vi "_Set_LO_frq_B10_WCA.vi"(1 "Bias_LO_equip":T1={"Node address"=19, "CAN Interface"="CAN0", "Cartridge band"=10, "Slave Node in"={"Address"=19, "Serial Number"=[16, 71, 55, 76, 1, 8, 0, -15]}, "ObjHandle out"=288096320, "POL"=0, "sb"=1, "GPIB_SM (SIS S,V)"="24", "GPIB_DMM (SIS I)"="22", "GPIB_SM (MAG I) "="25", "GPIB_SG(LO)"="19", "GPIB_PW (PAMP) "="6", "GPIB_TMP1(8ch)"="12", "GPIB_TMP2(2ch)  "="13", "WCA_avg"=10, "Rsen"=10.0, "BiasModule"=1, "LOModule "=2, "WCA_LO_FREQ_SET"={"YTO Low freq. [GHz]"=14.41, "YTO High freq. [GHz]"=17.71, "Kvco"=1, "Lock Pol."=0, "SET LO FREQ"=96.22222, "Multiplier"=6.0, "YTO (HEX)"=2015, "YTO ( FREQ)"=16.03381, "NULL PLL INTEGRATOR"=FALSE}, "Res for"=0} {"Res for" items=["none", "series res", "parallel res"]; "WCA_LO_FREQ_SET"."YTO ( FREQ)" min=25 max=150 step=0.0001 format="%.3f"; "WCA_LO_FREQ_SET"."Multiplier" min=3 max=6 step=3; "WCA_LO_FREQ_SET"."SET LO FREQ" min=25 max=150 step=0.0001 format="%.3f"; "WCA_LO_FREQ_SET"."Lock Pol." items=["Lower", "Upper"]; "WCA_LO_FREQ_SET"."Kvco" items=["7.5MHz/V", "15MHz/V"]; "WCA_LO_FREQ_SET"."YTO High freq. [GHz]" format="%.3f"; "WCA_LO_FREQ_SET"."YTO Low freq. [GHz]" format="%.3f"; "LOModule" items=["Manual Gunn+PAMP"=0, "PLL GUNN+PAMP"=5, "B10Lab LO"=1, "WCA LO"=2, ""=3, "YIG発信器"=4, "none"=99]; "BiasModule" items=["B10Lab Bias"=0, "WCA BiasModule"=1, "none"=99]; "Slave Node in"."Serial Number" format="%.0x"; "Slave Node in"."Address" format="%.0x"; "Cartridge band" max=10 step=1; "Node address" format="%.0x"}, 2 "LO_misc":T2={"LO FRQ(GHz)"=860.0, "LO multi "=9.0, "LocK?"=TRUE, "LO REF multi"=4.0, "wait (ms)"=100.0, "SG Pow Min (dBm)"=10.0, "SG Pow Max (dBm)"=20.0, "SG Pow Step (dBm)"=0.2, "SGPow OPT? "=TRUE, "SG set frq"=23.89638888888889, "SG set pow"=10.0}, 5 "error in (no error)":errorcluster) -> (14 "Bias_LO_equip 2":T1={"Node address"=19, "CAN Interface"="CAN0", "Cartridge band"=10, "Slave Node in"={"Address"=0, "Serial Number"=[]}, "ObjHandle out"=0, "POL"=1, "sb"=1, "GPIB_SM (SIS S,V)"="24", "GPIB_DMM (SIS I)"="22", "GPIB_SM (MAG I) "="25", "GPIB_SG(LO)"="19", "GPIB_PW (PAMP) "="6", "GPIB_TMP1(8ch)"="12", "GPIB_TMP2(2ch)  "="13", "WCA_avg"=10, "Rsen"=10.0, "BiasModule"=1, "LOModule "=1, "WCA_LO_FREQ_SET"={"YTO Low freq. [GHz]"=14.42, "YTO High freq. [GHz]"=17.7, "Kvco"=1, "Lock Pol."=0, "SET LO FREQ"=72.5, "Multiplier"=6.0, "YTO (HEX)"=0, "YTO ( FREQ)"=25.0, "NULL PLL INTEGRATOR"=FALSE}, "Res for"=0} {"Res for" items=["none", "series res", "parallel res"]; "WCA_LO_FREQ_SET"."YTO ( FREQ)" min=25 max=150 step=0.0001 format="%.4f"; "WCA_LO_FREQ_SET"."Multiplier" min=3 max=6 step=3; "WCA_LO_FREQ_SET"."SET LO FREQ" min=25 max=150 step=0.0001 format="%.3f"; "WCA_LO_FREQ_SET"."Lock Pol." items=["Lower", "Upper"]; "WCA_LO_FREQ_SET"."Kvco" items=["7.5MHz/V", "15MHz/V"]; "WCA_LO_FREQ_SET"."YTO High freq. [GHz]" format="%.3f"; "WCA_LO_FREQ_SET"."YTO Low freq. [GHz]" format="%.3f"; "LOModule" items=["Manual", "B10Lab LO", "WCA LO"]; "BiasModule" items=["B10Lab Bias", "WCA BiasModule"]; "Slave Node in"."Serial Number" format="%.0x"; "Slave Node in"."Address" format="%.0x"; "Cartridge band" max=10 step=1; "Node address" format="%.0x"}, 16 "LO_misc 2":T2={"LO FRQ(GHz)"=860.0, "LO multi "=9.0, "LocK?"=TRUE, "LO REF multi"=4.0, "wait (ms)"=100.0, "SG Pow Min (dBm)"=10.0, "SG Pow Max (dBm)"=20.0, "SG Pow Step (dBm)"=0.2, "SGPow OPT? "=TRUE, "SG set frq"=23.89638888888889, "SG set pow"=10.0}, 19 "error out":errorcluster)   [LabVIEW 2017]
uses:
  WCA_NAOJ_sub_vi/WCA_Global.vi
panel:
  # "LO freq. [GHz]"
  # "YTO LOW\n/High Freq."
  # "ZERO Intgrtr"
  # "Node Address"
  # "Serial Number"
  # "LO freq. [GHz]"
  # "YTO LOW\n/High Freq."
  # "ZERO Intgrtr"
  # "Node Address"
  # "Serial Number"
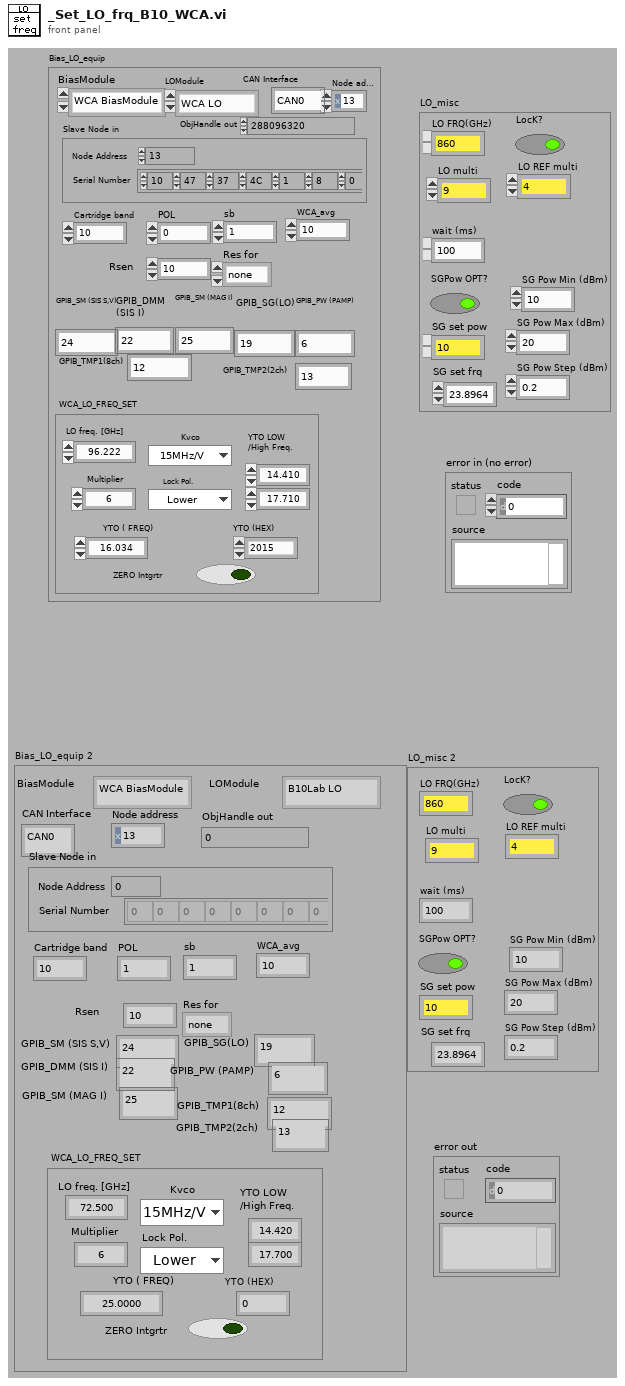
[diagram p1: front panel]
types:
  T1 = cluster{"Node address":u16, "CAN Interface":string, "Cartridge band":u32, "Slave Node in":cluster{"Address":i16, "Serial Number":i8[]}, "ObjHandle out":u32, "POL":u32, "sb":u32, "GPIB_SM (SIS S,V)":string, "GPIB_DMM (SIS I)":string, "GPIB_SM (MAG I) ":string, "GPIB_SG(LO)":string, "GPIB_PW (PAMP) ":string, "GPIB_TMP1(8ch)":string, "GPIB_TMP2(2ch)  ":string, "WCA_avg":i32, "Rsen":dbl, "BiasModule":u16, "LOModule ":u16, "WCA_LO_FREQ_SET":cluster{"YTO Low freq. [GHz]":sgl, "YTO High freq. [GHz]":sgl, "Kvco":u16, "Lock Pol.":u16, "SET LO FREQ":sgl, "Multiplier":sgl, "YTO (HEX)":u16, "YTO ( FREQ)":sgl, "NULL PLL INTEGRATOR":bool}, "Res for":u16}
  T2 = cluster{"LO FRQ(GHz)":dbl, "LO multi ":dbl, "LocK?":bool, "LO REF multi":dbl, "wait (ms)":dbl, "SG Pow Min (dBm)":dbl, "SG Pow Max (dBm)":dbl, "SG Pow Step (dBm)":dbl, "SGPow OPT? ":bool, "SG set frq":dbl, "SG set pow":dbl}
  T3 = cluster{"YTO Low freq. [GHz]":sgl, "YTO High freq. [GHz]":sgl, "Kvco":u16, "Lock Pol.":u16, "SET LO FREQ":sgl, "Multiplier":sgl, "YTO (HEX)":u16, "YTO ( FREQ)":sgl, "NULL PLL INTEGRATOR":bool}
  T4 = cluster{"YTO Low freq. [GHz]":sgl, "YTO High freq. [GHz]":sgl, "Kvco":u16, "Lock Pol.":u16, "SET LO FREQ":sgl, "Multiplier":sgl, "YTO coarse tune(HEX)":u16, "YTO coarse( FREQ)":sgl, "NULL PLL INTEGRATOR":bool}
  T5 = cluster{"PLL_ASSY_T":sgl, "PLL_REF_TOT_P":sgl, "PLL_IF_TOT_P":sgl, "PLL_CORR_V":sgl, "PLL_LOCK_V":sgl, "PLL_5V_SUPPLY_V":sgl, "Temp_TF":bool, "PLL Ref Pwr_TF":bool, "IF Pwr_TF":bool, "PLL Corr_TF":bool, "PLL Lock V_TF":bool, "PLL Nominal_TF":bool}
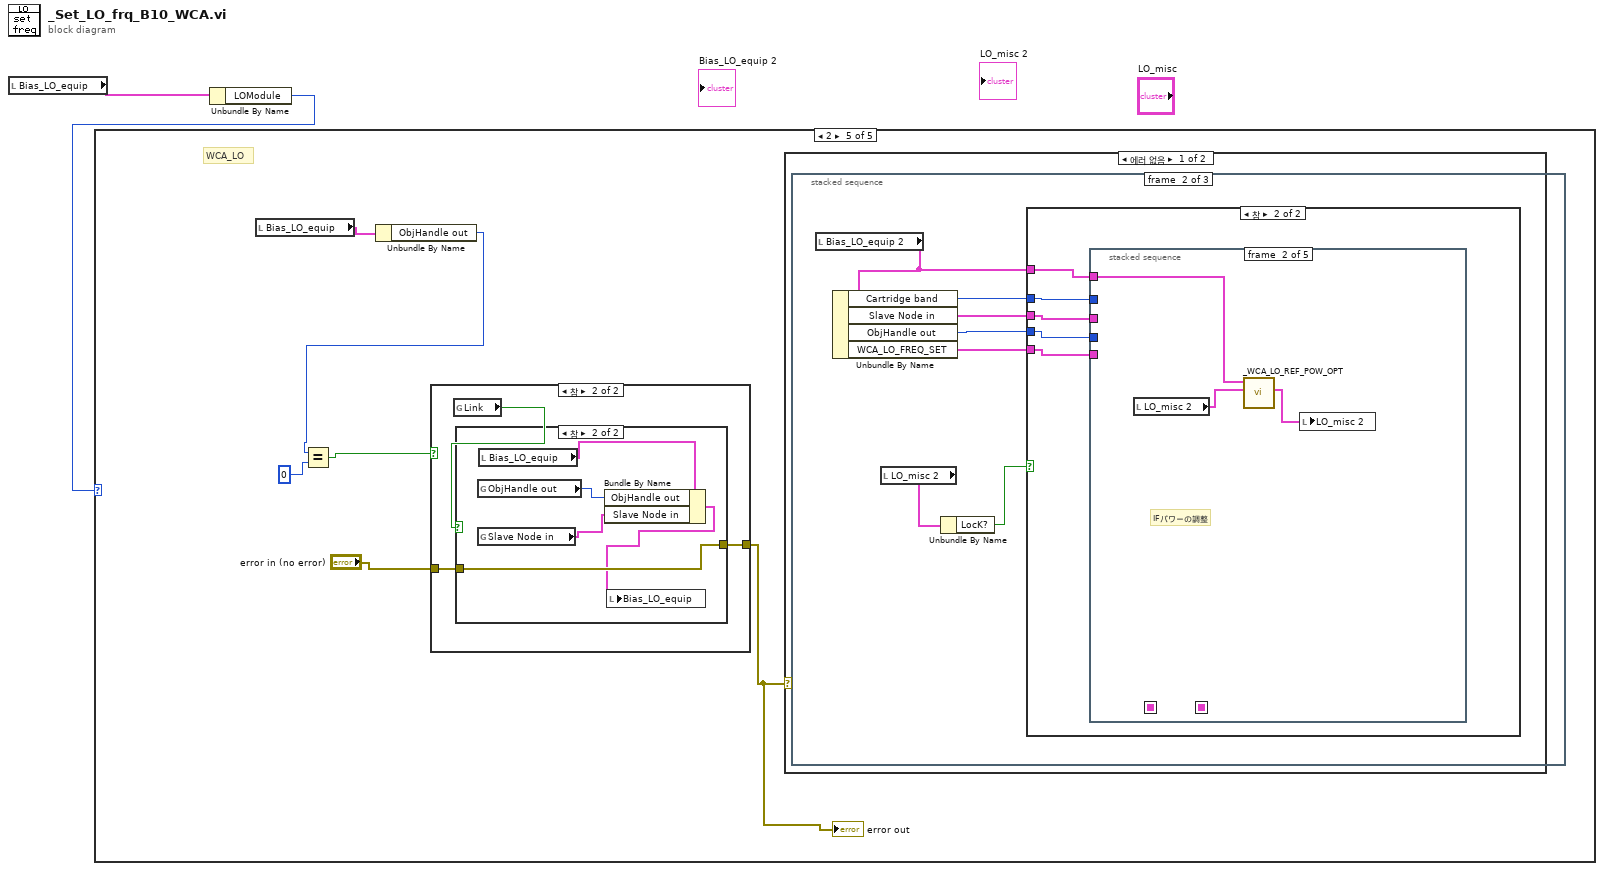
[diagram p0: block diagram]
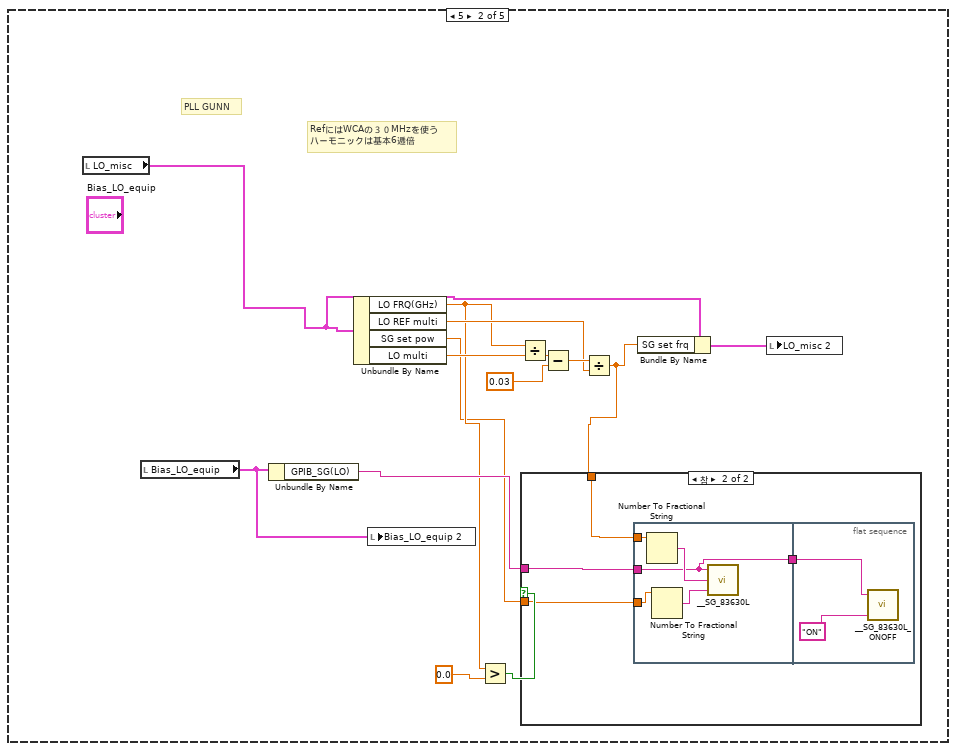
[diagram p3: hidden frame]
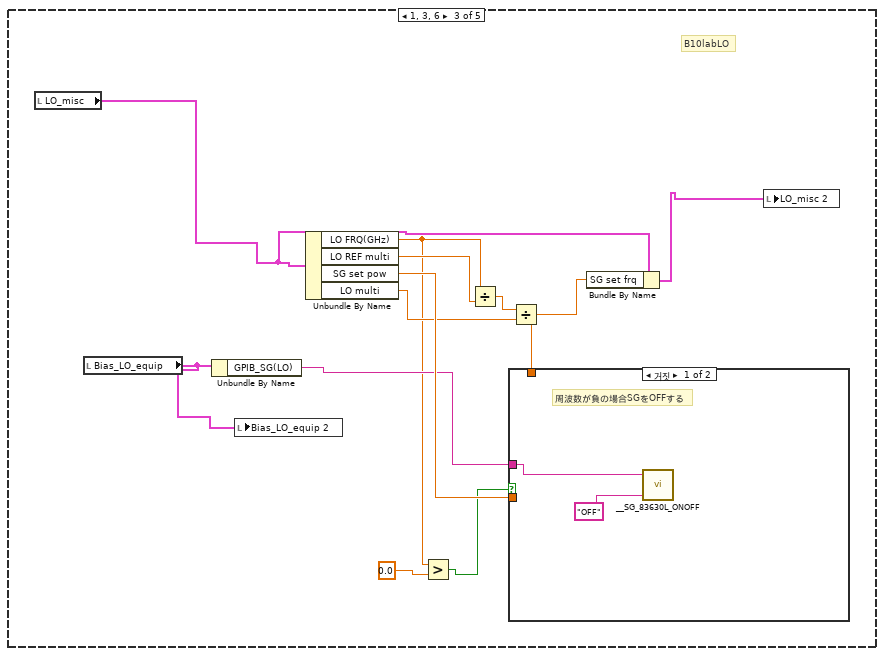
[diagram p5: hidden frame]
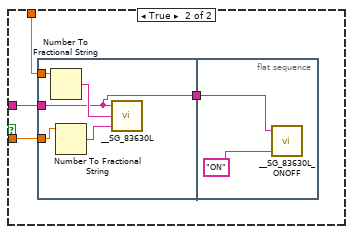
[diagram p6: hidden frame]
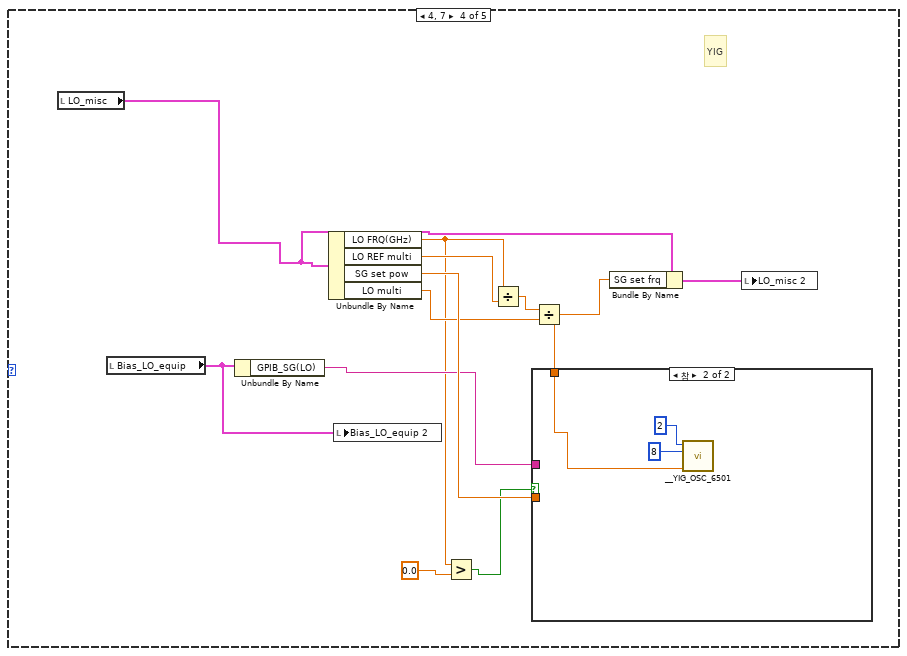
[diagram p7: hidden frame]
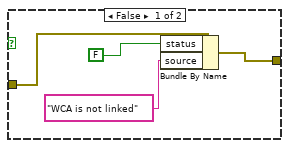
[diagram p10: hidden frame]
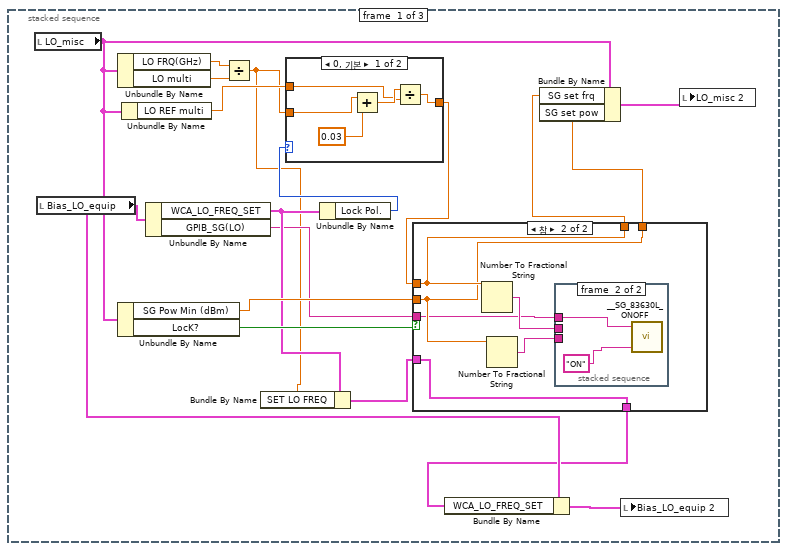
[diagram p11: hidden frame]
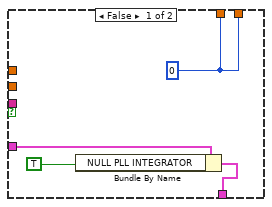
[diagram p12: hidden frame]
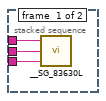
[diagram p13: hidden frame]
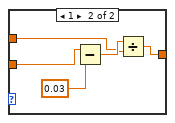
[diagram p14: hidden frame]
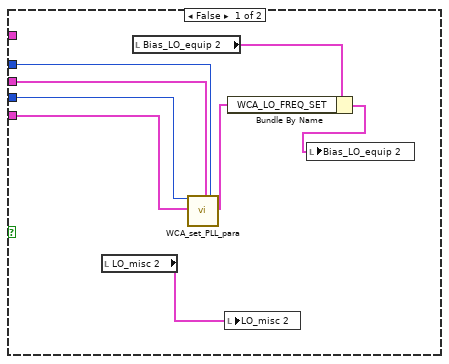
[diagram p15: hidden frame]
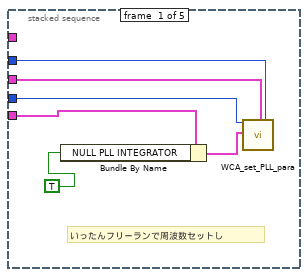
[diagram p16: hidden frame]
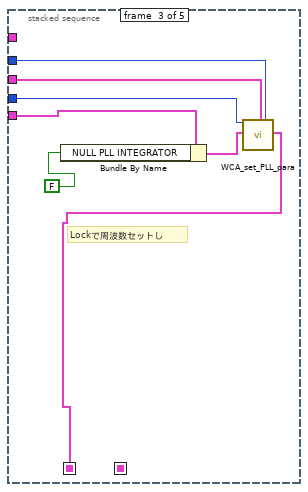
[diagram p17: hidden frame]
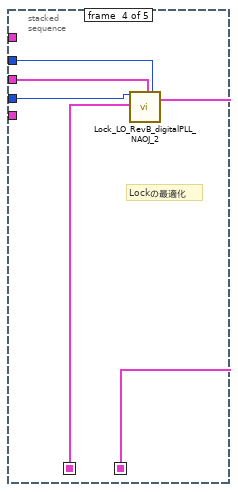
[diagram p18: hidden frame]
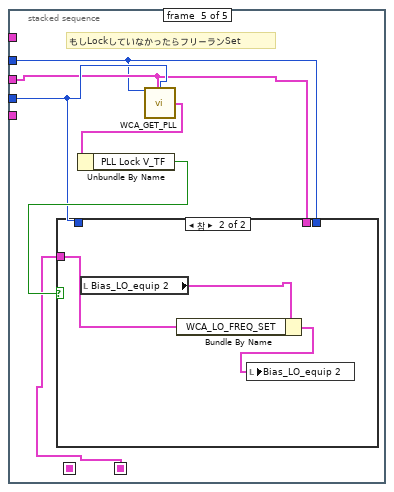
[diagram p19: hidden frame]
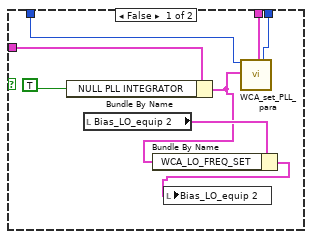
[diagram p20: hidden frame]
diagram:
  n1 = local read "Bias_LO_equip"() -> (w1:T1)
  n2 = Unbundle By Name(w1) -> ("LOModule"=w2:u16)
  n3 = case shown="2" w2 {
    frame 0, Default {
      # "Gunn unLock"
    }
    frame 5 {
      # "RefにはWCAの３０MHzを使う\nハーモニックは基本6逓倍"
      # "PLL GUNN"
      n4 = local read "LO_misc"() -> (w16:T2)
      n5 = local read "Bias_LO_equip"() -> (w6:T1)
      n6 = Unbundle By Name(w6) -> ("GPIB_SG(LO)"=w9:string)
      n7 = Unbundle By Name(w16) -> ("LO FRQ(GHz)"=w5:dbl, "LO REF multi"=w10:dbl, "SG set pow"=w3:dbl, "LO multi"=w14:dbl)
      n8 = local write "Bias_LO_equip 2"(w6) -> ()
      n9 = Greater?(x=w5, y=0.0) -> (0:w7:bool)
      n10 = Divide(x=w5, y=w14) -> (x/y=w13:dbl)
      n11 = Subtract(x=w13, y=0.03) -> (x-y=w11:dbl)
      n12 = Divide(x=w11, y=w10) -> (x/y=w4:dbl)
      n13 = case shown="참" w7 {
        tunnel: w3 -> [_ w17]
        tunnel: w4 -> [_ w18]
        tunnel: w9 -> [_ w19]
        frame False {
        }
        frame True {
          n14 = flat-sequence {
            tunnel: w18 -> [w24]
            tunnel: w17 -> [w22]
            tunnel: w19 -> [w21]
            tunnel: [w21] -> w20
            tunnel: w20 -> [w26]
            frame #0 {
              n15 = Number To Fractional String(number=w24) -> (F-format string=w25:string)  [unwired: 3 in]
              n16 = Number To Fractional String(number=w22) -> (F-format string=w23:string)  [unwired: 3 in]
              n17 = call "__SG_83630L.vi"("PW(dBm)"=w23, "frq(GHz)"=w25, "GPIB"=w21) -> ()
            }
            frame #1 {
              n18 = call "__SG_83630L_ONOFF.vi"("ON/OFF"="ON", "GPIB"=w26) -> ()  [unwired: 1 in]
            }
          }
        }
      }
      n19 = Bundle By Name(cluster=w16, "SG set frq"=w4) -> (w15:T2)
      n20 = local write "LO_misc 2"(w15) -> ()
    }
    frame 1, 3, 6 {
      # "B10labLO"
      n21 = local read "LO_misc"() -> (w30:T2)
      n22 = local read "Bias_LO_equip"() -> (w28:T1)
      n23 = Unbundle By Name(w28) -> ("GPIB_SG(LO)"=w34:string)
      n24 = local write "Bias_LO_equip 2"(w28) -> ()
      n25 = Unbundle By Name(w30) -> ("LO FRQ(GHz)"=w32:dbl, "LO REF multi"=w38:dbl, "SG set pow"=w37:dbl, "LO multi"=w35:dbl)
      n26 = Greater?(x=w32, y=0.0) -> (0:w31:bool)
      n27 = Divide(x=w32, y=w38) -> (x/y=w39:dbl)
      n28 = Divide(x=w39, y=w35) -> (x/y=w36:dbl)
      n29 = case shown="거짓" w31 {
        tunnel: w37 -> [_ w44]
        tunnel: w36 -> [_ w43]
        tunnel: w34 -> [w40 w42]
        frame False {
          # "周波数が負の場合SGをOFFする"
          n30 = call "__SG_83630L_ONOFF.vi"("ON/OFF"="OFF", "GPIB"=w40) -> ()  [unwired: 1 in]
        }
        frame True {
          n31 = flat-sequence {
            tunnel: w43 -> [w49]
            tunnel: w44 -> [w47]
            tunnel: w42 -> [w46]
            tunnel: [w46] -> w45
            tunnel: w45 -> [w51]
            frame #0 {
              n32 = Number To Fractional String(number=w49) -> (F-format string=w50:string)  [unwired: 3 in]
              n33 = Number To Fractional String(number=w47) -> (F-format string=w48:string)  [unwired: 3 in]
              n34 = call "__SG_83630L.vi"("PW(dBm)"=w48, "frq(GHz)"=w50, "GPIB"=w46) -> ()
            }
            frame #1 {
              n35 = call "__SG_83630L_ONOFF.vi"("ON/OFF"="ON", "GPIB"=w51) -> ()  [unwired: 1 in]
            }
          }
        }
      }
      n36 = Bundle By Name(cluster=w30, "SG set frq"=w36) -> (w29:T2)
      n37 = local write "LO_misc 2"(w29) -> ()
    }
    frame 4, 7 {
      # "YIG"
      n38 = local read "LO_misc"() -> (w55:T2)
      n39 = local read "Bias_LO_equip"() -> (w54:T1)
      n40 = Unbundle By Name(w54) -> ("GPIB_SG(LO)"=w59:string)
      n41 = Unbundle By Name(w55) -> ("LO FRQ(GHz)"=w57:dbl, "LO REF multi"=w63:dbl, "SG set pow"=w62:dbl, "LO multi"=w60:dbl)
      n42 = local write "Bias_LO_equip 2"(w54) -> ()
      n43 = Greater?(x=w57, y=0.0) -> (0:w56:bool)
      n44 = Divide(x=w57, y=w63) -> (x/y=w64:dbl)
      n45 = Divide(x=w64, y=w60) -> (x/y=w61:dbl)
      n46 = case shown="참" w56 {
        tunnel: w62 -> [_ _]
        tunnel: w61 -> [_ w65]
        tunnel: w59 -> [_ _]
        frame False {
        }
        frame True {
          n47 = call "__YIG_OSC_6501.vi"("fc(GHz)"=w65, "bit"=8, "Dev(1,2..)"=2) -> ()  [unwired: 1 in]
        }
      }
      n48 = Bundle By Name(cluster=w55, "SG set frq"=w61) -> (w53:T2)
      n49 = local write "LO_misc 2"(w53) -> ()
    }
    frame 2 {
      # "WCA_LO"
      n50 = local read "Bias_LO_equip"() -> (w70:T1)
      n51 = Unbundle By Name(w70) -> ("ObjHandle out"=w69:u32)
      n52 = Equal?(x=w69, y=0) -> (x = y?=w72:bool)
      n53 = case shown="참" w72 {
        tunnel: "error in (no error)" -> [w74 w77]
        tunnel: [w74 w76] -> w68
        frame False {
        }
        frame True {
          n54 = global read "WCA_Global.vi" "Link"() -> (w75:bool)
          n55 = case shown="참" w75 {
            tunnel: w77 -> [w81 w86]
            tunnel: [w78 w86] -> w76
            frame False {
              n56 = Bundle By Name(cluster=w81, "status"=FALSE, "source"="WCA is not linked") -> (w78:errorcluster)
            }
            frame True {
              n57 = global read "WCA_Global.vi" "ObjHandle out"() -> (w83:u32)
              n58 = global read "WCA_Global.vi" "Slave Node in"() -> (w84:cluster{"Address":i16, "Serial Number":i8[]})
              n59 = local read "Bias_LO_equip"() -> (w85:T1)
              n60 = Bundle By Name(cluster=w85, "ObjHandle out"=w83, "Slave Node in"=w84) -> (w82:T1)
              n61 = local write "Bias_LO_equip"(w82) -> ()
            }
          }
        }
      }
      "error out" <- w68
      n62 = case shown="에러 없음" w68 {
        frame No Error {
          n63 = stacked-sequence {
            frame #0 {
              n64 = local read "LO_misc"() -> (w103:T2)
              n65 = local read "Bias_LO_equip"() -> (w91:T1)
              n66 = Unbundle By Name(w103) -> ("LO FRQ(GHz)"=w101:dbl, "LO multi"=w102:dbl)
              n67 = Unbundle By Name(w103) -> ("SG Pow Min (dBm)"=w97:dbl, "LocK?"=w96:bool)
              n68 = Unbundle By Name(w103) -> ("LO REF multi"=w100:dbl)
              n69 = Unbundle By Name(w91) -> ("WCA_LO_FREQ_SET"=w94:T3, "GPIB_SG(LO)"=w93:string)
              n70 = Divide(x=w101, y=w102) -> (x/y=w92:dbl)
              n71 = Bundle By Name(cluster=w94, "SET LO FREQ"=w92) -> (w95:T3)
              n72 = Unbundle By Name(w94) -> ("Lock Pol."=w99:u16)
              n73 = case shown="0, 기본" w99 {
                tunnel: w92 -> [w124 w129]
                tunnel: w100 -> [w121 w126]
                tunnel: [w120 w125] -> w98
                frame 0, Default {
                  n74 = Add(x=w124, y=0.03) -> (x+y=w122:dbl)
                  n75 = Divide(x=w122, y=w121) -> (x/y=w120:dbl)
                }
                frame 1 {
                  n76 = Subtract(x=w129, y=0.03) -> (x-y=w127:dbl)
                  n77 = Divide(x=w127, y=w126) -> (x/y=w125:dbl)
                }
              }
              n78 = case shown="참" w96 {
                tunnel: w98 -> [_ w111]
                tunnel: w97 -> [_ w110]
                tunnel: w93 -> [_ w109]
                tunnel: w95 -> [w108 w112]
                tunnel: [w107 w112] -> w90
                tunnel: [w105 w111] -> w88
                tunnel: [w105 w110] -> w87
                frame False {
                  w105 = 0
                  n79 = Bundle By Name(cluster=w108, "NULL PLL INTEGRATOR"=TRUE) -> (w107:T3)
                }
                frame True {
                  n80 = Number To Fractional String(number=w111) -> (F-format string=w113:string)  [unwired: 3 in]
                  n81 = Number To Fractional String(number=w110) -> (F-format string=w114:string)  [unwired: 3 in]
                  n82 = stacked-sequence {
                    tunnel: w114 -> [w117 _]
                    tunnel: w113 -> [w116 _]
                    tunnel: w109 -> [w115 w119]
                    frame #0 {
                      n83 = call "__SG_83630L.vi"("PW(dBm)"=w117, "frq(GHz)"=w116, "GPIB"=w115) -> ()
                    }
                    frame #1 {
                      n84 = call "__SG_83630L_ONOFF.vi"("ON/OFF"="ON", "GPIB"=w119) -> ()  [unwired: 1 in]
                    }
                  }
                }
              }
              n85 = Bundle By Name(cluster=w91, "WCA_LO_FREQ_SET"=w90) -> (w89:T1)
              n86 = Bundle By Name(cluster=w103, "SG set frq"=w88, "SG set pow"=w87) -> (w104:T2)
              n87 = local write "Bias_LO_equip 2"(w89) -> ()
              n88 = local write "LO_misc 2"(w104) -> ()
            }
            frame #1 {
              n89 = local read "Bias_LO_equip 2"() -> (w130:T1)
              n90 = Unbundle By Name(w130) -> ("Cartridge band"=w132:u32, "Slave Node in"=w134:cluster{"Address":i16, "Serial Number":i8[]}, "ObjHandle out"=w133:u32, "WCA_LO_FREQ_SET"=w131:T3)
              n91 = local read "LO_misc 2"() -> (w135:T2)
              n92 = Unbundle By Name(w135) -> ("LocK?"=w136:bool)
              n93 = case shown="참" w136 {
                tunnel: w134 -> [w144 w147]
                tunnel: w133 -> [w141 w148]
                tunnel: w132 -> [w143 w146]
                tunnel: w131 -> [w142 w149]
                tunnel: w130 -> [_ w145]
                frame False {
                  n94 = local read "LO_misc 2"() -> (w137:T2)
                  n95 = local read "Bias_LO_equip 2"() -> (w140:T1)
                  n96 = call "WCA_set_PLL_para.vi"("ObjHandle in"=w141, "LO_FREQ_SET"=w142, "Slave Node in"=w144, "Cartridge band"=w143) -> ("LO_FREQ_SET output"=w138:T4)  [unwired: 14 in, 1 out]
                  n97 = local write "LO_misc 2"(w137) -> ()
                  n98 = Bundle By Name(cluster=w140, "WCA_LO_FREQ_SET"=w138) -> (w139:T1)
                  n99 = local write "Bias_LO_equip 2"(w139) -> ()
                }
                frame True {
                  n100 = stacked-sequence {
                    seq-local: [_ _ w159 _ _] -> [_ _ _ w170 _]
                    seq-local: [_ _ _ w166 _] -> [_ _ _ _ w171]
                    tunnel: w149 -> [w155 _ w165 _ _]
                    tunnel: w148 -> [w152 _ w162 w169 w174]
                    tunnel: w147 -> [w151 _ w161 w168 w173]
                    tunnel: w146 -> [w150 _ w160 w167 w172]
                    tunnel: w145 -> [_ w156 _ _ _]
                    frame #0 {
                      # "いったんフリーランで周波数セットし"
                      n101 = Bundle By Name(cluster=w155, "NULL PLL INTEGRATOR"=TRUE) -> (w153:T3)
                      n102 = call "WCA_set_PLL_para.vi"("ObjHandle in"=w152, "LO_FREQ_SET"=w153, "Slave Node in"=w151, "Cartridge band"=w150) -> ()  [unwired: 14 in, 2 out]
                    }
                    frame #1 {
                      # "IFパワーの調整"
                      n103 = local read "LO_misc 2"() -> (w158:T2)
                      n104 = call "_WCA_LO_REF_POW_OPT.vi"("LO_misc"=w158, "Bias_LO_equip"=w156) -> ("LO_misc 2"=w157:T2)  [unwired: 6 in, 1 out]
                      n105 = local write "LO_misc 2"(w157) -> ()
                    }
                    frame #2 {
                      # "Lockで周波数セットし"
                      n106 = Bundle By Name(cluster=w165, "NULL PLL INTEGRATOR"=FALSE) -> (w163:T3)
                      n107 = call "WCA_set_PLL_para.vi"("ObjHandle in"=w162, "LO_FREQ_SET"=w163, "Slave Node in"=w161, "Cartridge band"=w160) -> ("LO_FREQ_SET output"=w159:T4)  [unwired: 14 in, 1 out]
                    }
                    frame #3 {
                      # "Lockの最適化"
                      n108 = call "Lock_LO_RevB_digitalPLL_NAOJ_2.vi"("ObjHandle in"=w169, "LO_FREQ_SET"=w170, "Slave Node in"=w168, "Cartridge band"=w167) -> ("LO_FREQ_output"=w166:T4)  [unwired: 12 in, 3 out]
                    }
                    frame #4 {
                      # "もしLockしていなかったらフリーランSet"
                      n109 = call "WCA_GET_PLL.vi"("Cartridge Band"=w172, "Slave Node in"=w173, "ObjHandle in"=w174) -> ("GET_PLL"=w176:T5)  [unwired: 10 in, 2 out]
                      n110 = Unbundle By Name(w176) -> ("PLL Lock V_TF"=w175:bool)
                      n111 = case shown="참" w175 {
                        tunnel: w171 -> [w183 w185]
                        tunnel: w174 -> [w182 _]
                        tunnel: w173 -> [w181 _]
                        tunnel: w172 -> [w180 _]
                        frame False {
                          n112 = Bundle By Name(cluster=w183, "NULL PLL INTEGRATOR"=TRUE) -> (w178:T4)
                          n113 = local read "Bias_LO_equip 2"() -> (w179:T1)
                          n114 = Bundle By Name(cluster=w179, "WCA_LO_FREQ_SET"=w178) -> (w177:T1)
                          n115 = local write "Bias_LO_equip 2"(w177) -> ()
                          n116 = call "WCA_set_PLL_para.vi"("ObjHandle in"=w182, "LO_FREQ_SET"=w178, "Slave Node in"=w181, "Cartridge band"=w180) -> ()  [unwired: 14 in, 2 out]
                        }
                        frame True {
                          n117 = local read "Bias_LO_equip 2"() -> (w187:T1)
                          n118 = Bundle By Name(cluster=w187, "WCA_LO_FREQ_SET"=w185) -> (w186:T1)
                          n119 = local write "Bias_LO_equip 2"(w186) -> ()
                        }
                      }
                    }
                  }
                }
              }
            }
            frame #2 {
              n120 = local read "Bias_LO_equip 2"() -> (w189:T1)
              n121 = Unbundle By Name(w189) -> ("ObjHandle out"=w196:u32, "Slave Node in"=w195:cluster{"Address":i16, "Serial Number":i8[]}, "Cartridge band"=w194:u32, "WCA_LO_FREQ_SET.YTO Low freq. [GHz]"=w192:sgl, "WCA_LO_FREQ_SET.YTO High freq. [GHz]"=w193:sgl)
              n122 = call "YTO_Read_Coarse_tune_Naoj.vi"("Cartridge band"=w194, "Slave Node in"=w195, "ObjHandle in"=w196) -> ("YTO Coarse Tune"=w191:u16)  [unwired: 6 in, 2 out]
              n123 = call "LO_YTO-count2freq_naoj.vi"("f max"=w193, "f min"=w192, "YTO count"=w191) -> ("YTO freq."=w190:sgl)  [unwired: 6 in]
              n124 = Bundle By Name(cluster=w189, "WCA_LO_FREQ_SET.YTO (HEX)"=w191, "WCA_LO_FREQ_SET.YTO ( FREQ)"=w190) -> (w188:T1)
              n125 = local write "Bias_LO_equip 2"(w188) -> ()
            }
          }
        }
        frame Error {
          (unwired) sgl -1.0 ("SET YTO COARSE TUNE")
        }
      }
    }
  }
